vi "DT2_discrete_b2.vi"(8 "error in (no error)":errorcluster, 9 "f0":dbl, 10 "Tcyc":dbl, 11 "D":dbl) -> (0 "error out":errorcluster, 3 "b2":dbl)   [LabVIEW 2022 SP3]
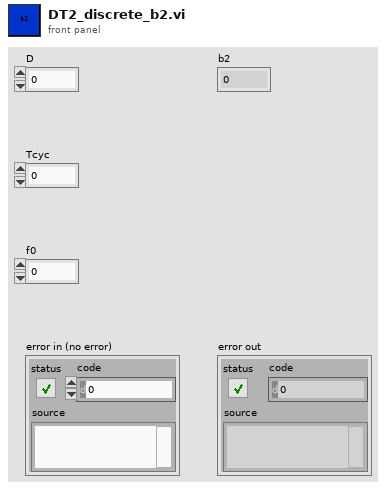
[diagram p1: front panel]
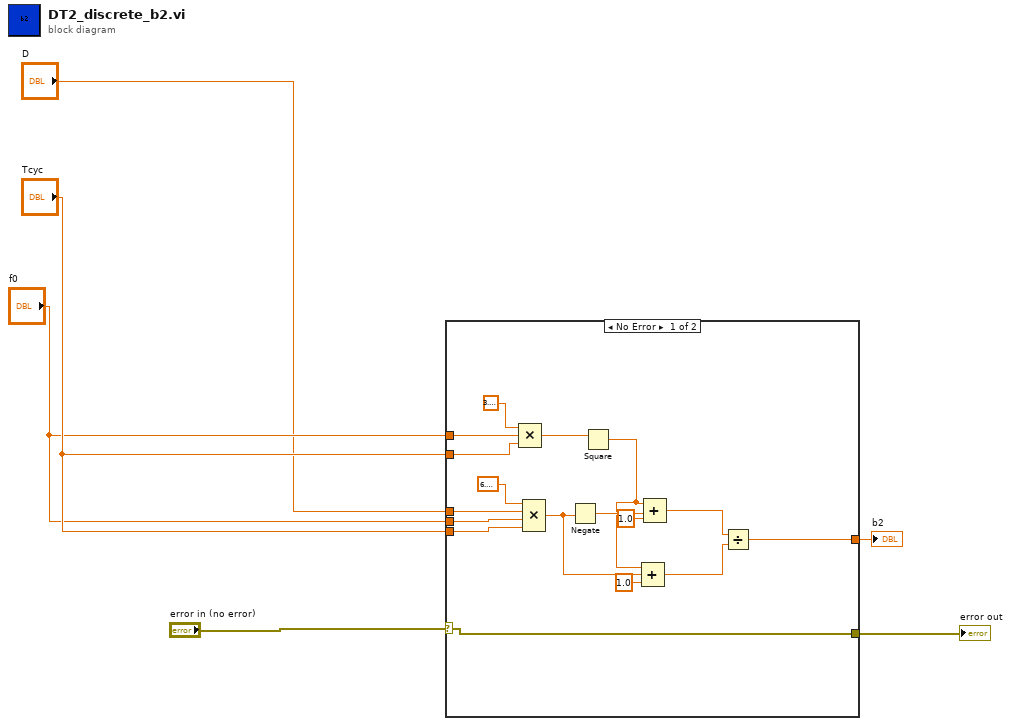
[diagram p0: block diagram]
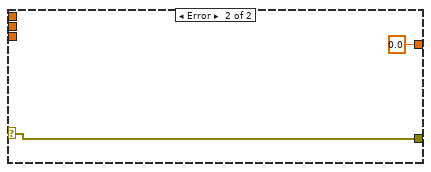
[diagram p2: hidden frame]
diagram:
  n1 = case shown="No Error" "error in (no error)" {
    selector: "error in (no error)" -> [w7 w24]
    tunnel: "f0" -> [w22 _]
    tunnel: "Tcyc" -> [w21 _]
    tunnel: "D" -> [w18 _]
    tunnel: "f0" -> [w17 _]
    tunnel: "Tcyc" -> [w16 _]
    tunnel: [w8 0.0] -> w5
    tunnel: [w7 w24] -> w6
    frame No Error {
      n2 = Compound Arithmetic op=MULTIPLY(3.141592653589793, w22, w21) -> (w20:dbl)
      n3 = Compound Arithmetic op=MULTIPLY(6.283185307179586, w18, w17, w16) -> (w11:dbl)
      n4 = Negate(x=w11) -> (-x=w15:dbl)
      n5 = Square(x=w20) -> (x^2=w12:dbl)
      n6 = Compound Arithmetic op=ADD(w12, w11, 1.0 ("value")) -> (w9:dbl)
      n7 = Compound Arithmetic op=ADD(w12, w15, 1.0 ("value")) -> (w13:dbl)
      n8 = Divide(x=w13, y=w9) -> (x/y=w8:dbl)
    }
    frame Error {
    }
  }
  "error out" <- w6
  "b2" <- w5
